vi "Periodic Tasks.vi"(8 "error in":errorcluster) -> ()   [LabVIEW 2016]
doc: "This VI runs in parallel to other tasks. It can contain as many user-defined periodic loops as you need. These can carry out PID or other sorts of timed response."
uses:
  <vilib>/Rock Robotics/WPI/Utilities/WPI_GetSetVariantRefNum.vi
  <vilib>/Instr/_visa.llb/VISA Configure Serial Port (Instr).vi
  2_11_17/Systems/Global 1.vi
  <vilib>/Analysis/3filter.llb/IIR Filter (DBL).vi
  <vilib>/Analysis/NI_AALBase.lvlib
panel:
  in  "off set":dbl=55.0 format="%#_13g"
  out "read buffer":string="B:3,X:197.00,Y:124.00"
  in  "Search_Params":string[](array[string])=["B", "X", "Y", "W1", "H1", "W2", "H2"]
  out "Last Complete Message":string="B:2,X:197.00,Y:124.00,W1:9,H1:24,W2:9,H2:23"
  out "length":i32=43
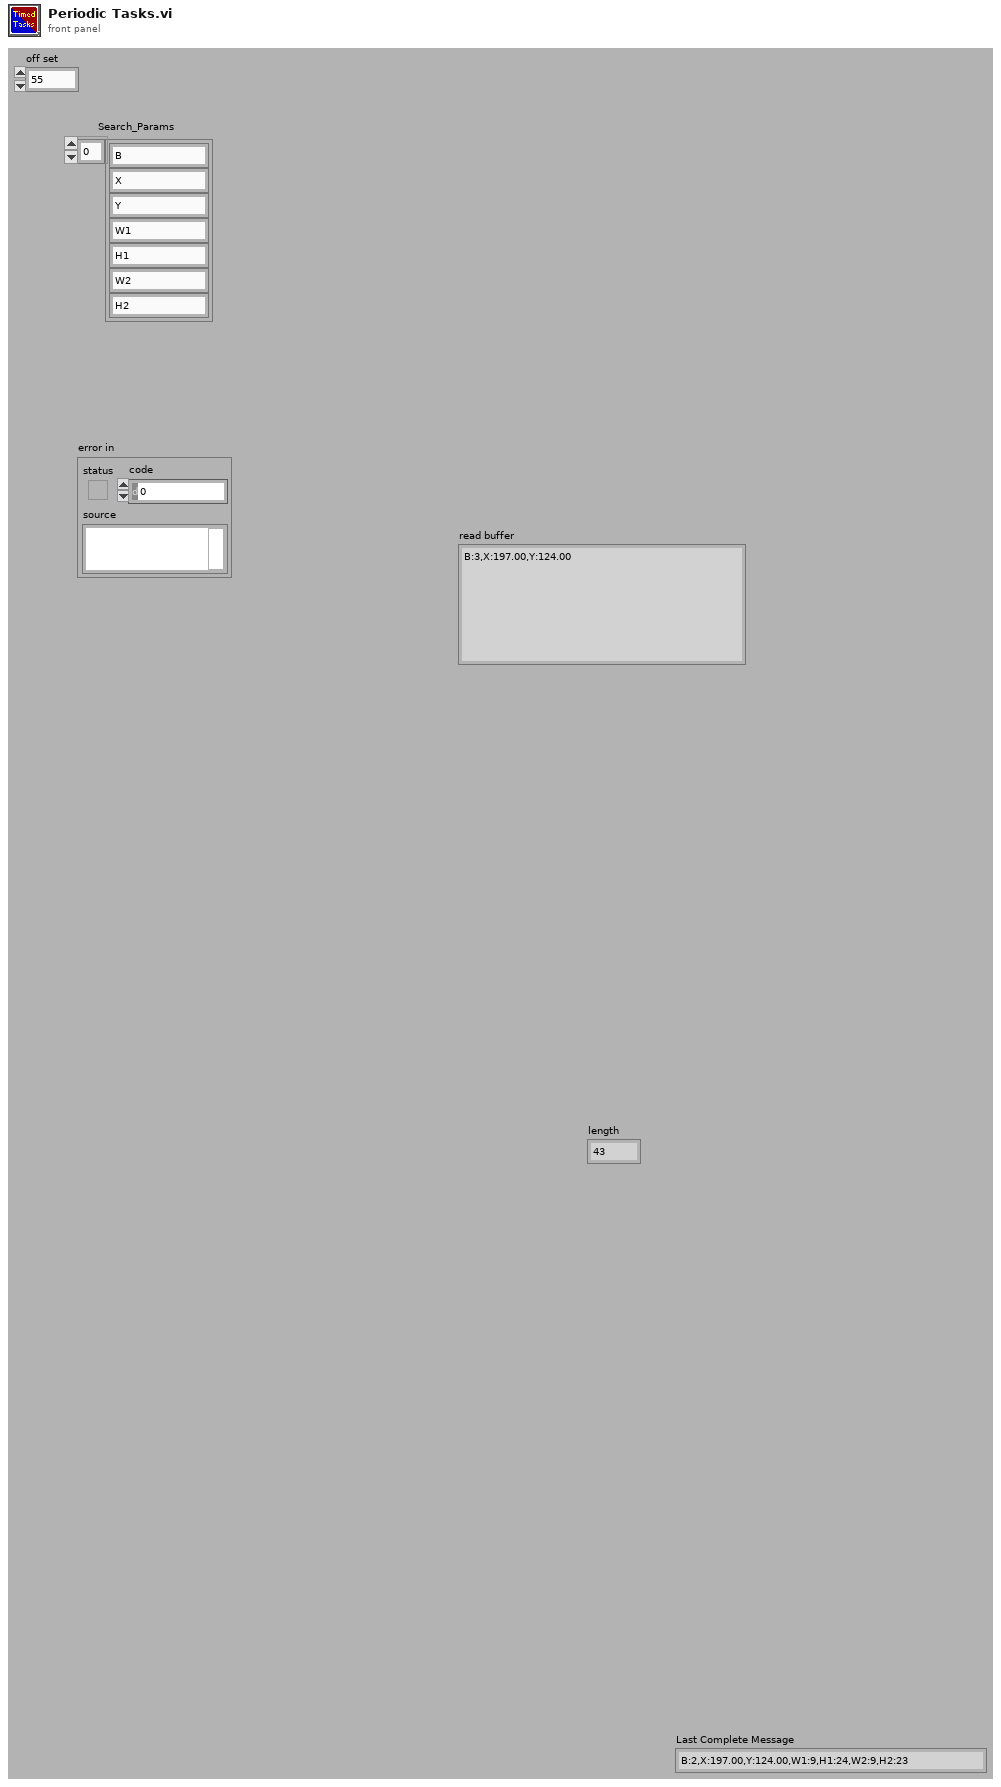
[diagram p1: front panel]
types:
  T1 = typedef "WPI_JoystickDevRef.ctl" = cluster{"Device":T2}
  T2 = typedef "WPI_JoystickDeviceEnum.ctl" = enum16{"USB 0", "USB 1", "USB 2", "USB 3", "USB 4", "USB 5"}
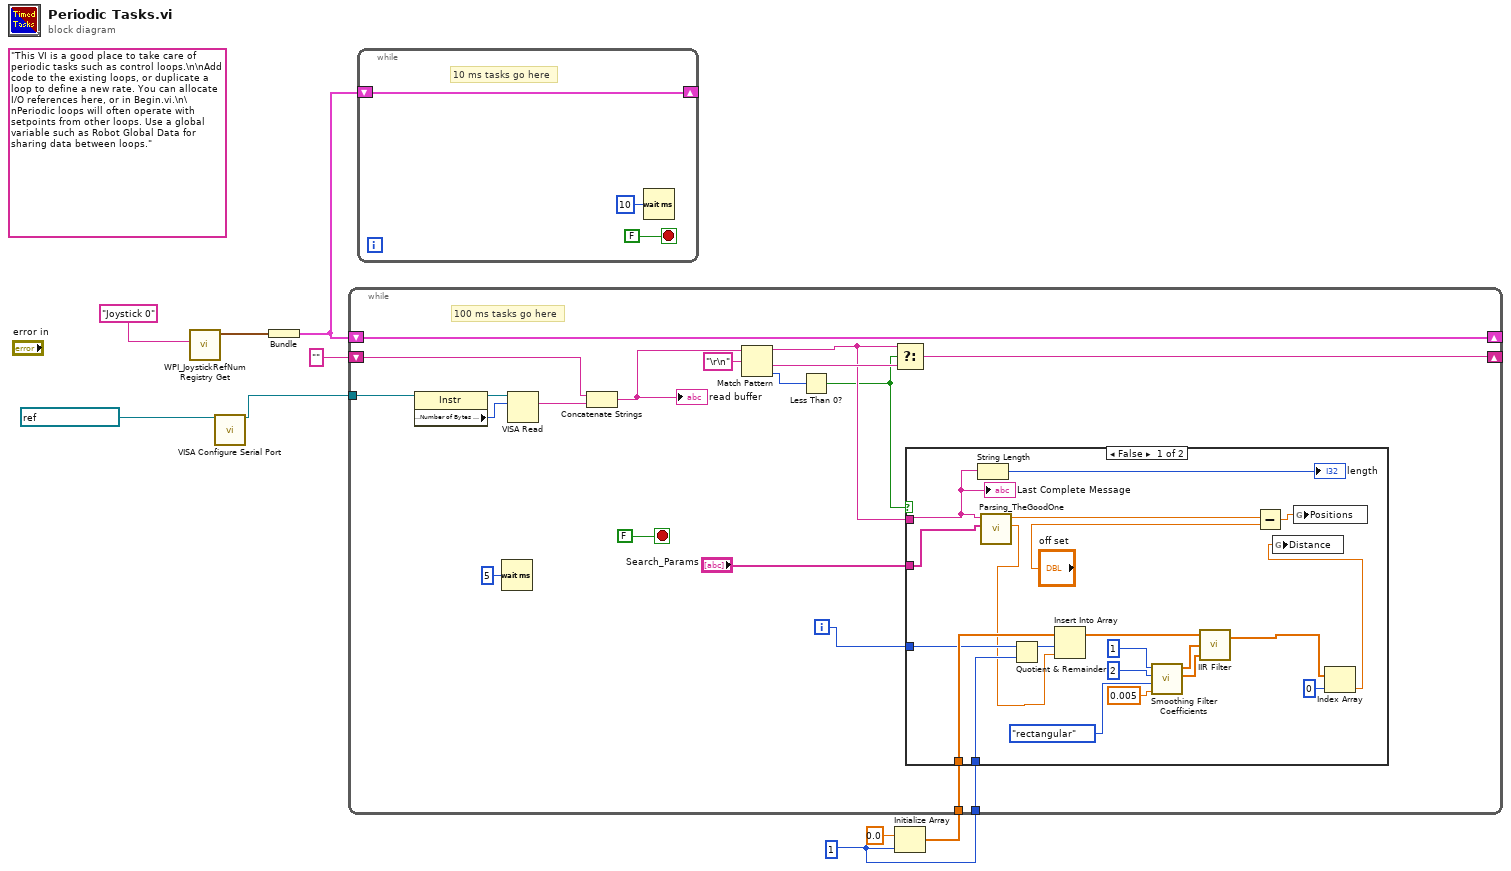
[diagram p0: block diagram]
diagram:
  w9 = 1
  (unwired) "This VI is a good place to take care of periodic tasks such as control loops.\n\nAdd code to the existing loops, or duplicate a loop to define a new rate. You can allocate I/O references here, or in Begin.vi.\n\nPeriodic loops will often operate with setpoints from other loops. Use a global variable such as Robot Global Data for sharing data between loops."
  n1 = call <vilib>:"WPI_JoystickRefNum Registry Get.vi"("refnum name"="Joystick 0") -> ("JoystickDevRef"=w5:T1)  [unwired: 1 in, 9 out]
  n2 = call-poly "VISA Configure Serial Port"("VISA resource name"=refnum<visa-resource-name> "ASRL2::INSTR") -> ("VISA resource name out"=w2:refnum<visa-resource-name>)  [unwired: 13 in, 1 out]
  n3 = Bundle("JoystickDevRef"=w5) -> (w4:cluster{"JoystickDevRef":T1})  [unwired: 1 out]
  n4 = while {
    shift-right: [w10] -> _
    shift-left: w4 -> [w10]
    stop <- FALSE stop-if-true
    # "10 ms tasks go here"
    n5 = Wait (ms)(milliseconds to wait=u32 10) -> ()  [unwired: 1 out]
  }
  n6 = Initialize Array(0.0 ("element"), w9) -> (w8:dbl[])
  n7 = while {
    shift-right: [w30] -> _
    shift-left: w4 -> [w30]
    tunnel: w2 -> [w25]
    shift-right: [w17] -> _
    shift-left: "" -> [w24]
    tunnel: w8 -> [w15]
    tunnel: w9 -> [w14]
    i -> [w13]
    stop <- FALSE stop-if-true
    # "100 ms tasks go here"
    n8 = property class="Instr"(reference=w25) -> (reference out=w29:refnum<visa-resource-name>, "Serial Settings:Number of Bytes at Serial Port"=w28:u32)  [unwired: 1 in, 1 out]
    n9 = Wait (ms)(milliseconds to wait=u32 5) -> ()  [unwired: 1 out]
    n10 = VISA Read(VISA resource name=w29, byte count=w28) -> (read buffer=w23:string)  [unwired: 1 in, 3 out]
    n11 = Concatenate Strings(w24, w23) -> (w22:string)
    "read buffer" <- w22
    n12 = Match Pattern(string=w22, regular expression="\r\n") -> (before substring=w18:string, after substring=w19:string, offset past match=w20:i32)  [unwired: 1 in, 1 out]
    n13 = Less Than 0?(x=w20) -> (x < 0?=w16:bool)
    n14 = Select(t=w18, s=w16, f=w19) -> (s? t:f=w17:string)
    n15 = case shown="False" w16 {
      tunnel: "Search_Params" -> [w51 _]
      tunnel: w18 -> [w50 _]
      tunnel: w15 -> [w38 _]
      tunnel: w14 -> [w37 _]
      tunnel: w13 -> [w36 _]
      frame False {
        n16 = String Length(string=w50) -> (length=→"length":i32)
        n17 = call "Parsing_TheGoodOne.vi"("Search_Params"=w51, "Input"=w50) -> ("Corrected distance"=w35:dbl, "Value-Reference"=w49:dbl)  [unwired: 6 in]
        n18 = Quotient & Remainder(x=w36, y=w37) -> (x-y*floor(x/y)=w39:i32)  [unwired: 1 out]
        n19 = Insert Into Array(array=w38, index=w39, new element=w35) -> (w40:dbl[])
        n20 = call <vilib>:"Smoothing Filter Coefficients.vi"("time constant"=0.005, "shape"=enum16{"rectangular", "triangular"}."rectangular", "half-width"=2, "type"=1) -> ("forward coefficients"=w42:dbl[], "reverse coefficients"=w43:dbl[])  [unwired: 5 in, 1 out]
        n21 = call-poly <vilib>:"IIR Filter.vi"("Forward Coefficients"=w42, "Reverse Coefficients"=w43, "X"=w40) -> ("Filtered X"=w34:dbl[])  [unwired: 1 in, 1 out]
        n22 = Subtract(x=w49, y="off set") -> (x-y=w47:dbl)
        n23 = global write "Global 1.vi" "Positions"(w47) -> ()
        n24 = Index Array(array=w34, index=0) -> (element=w32:dbl)
        n25 = global write "Global 1.vi" "Distance"(w32) -> ()
        "Last Complete Message" <- w50
      }
      frame True {
      }
    }
  }
